vi "10-Tap Conversion.vi"(8 "10 Tap In":T1, 9 "64 Bit In":u64, 10 "16 Bit In":u16, 11 "Operation":T2) -> (1 "10 Tap Out":T1, 2 "64 Bit Out":u64, 3 "16 Bit Out":u16)   [LabVIEW 2013]
uses:
  Common/CL Data to Pixels/10-Tap 8-bit Cluster.ctl
  10-Tap Conversion Enum.ctl
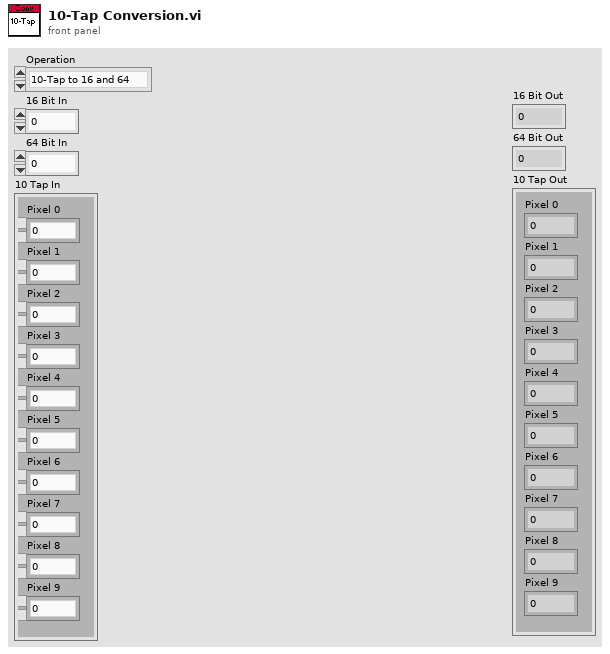
[diagram p1: front panel]
types:
  T1 = typedef "10-Tap 8-bit Cluster.ctl" = cluster{"Pixel 0":u8, "Pixel 1":u8, "Pixel 2":u8, "Pixel 3":u8, "Pixel 4":u8, "Pixel 5":u8, "Pixel 6":u8, "Pixel 7":u8, "Pixel 8":u8, "Pixel 9":u8}
  T2 = typedef "10-Tap Conversion Enum.ctl" = enum16{"10-Tap to 16 and 64", "16 and 64 to 10-Tap"}
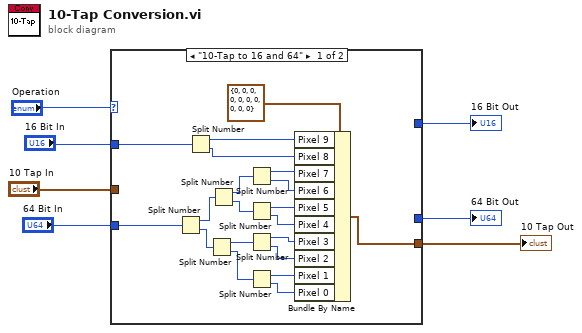
[diagram p0: block diagram]
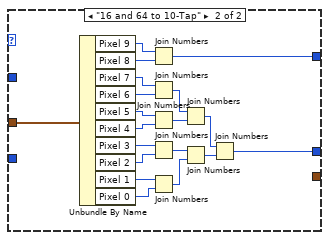
[diagram p2: hidden frame]
diagram:
  n1 = case shown="\"10-Tap to 16 and 64\"" "Operation" {
    tunnel: "10 Tap In" -> [_ w30]
    tunnel: [_ w29] -> w6
    tunnel: [_ w28] -> w5
    tunnel: "16 Bit In" -> [w10 _]
    tunnel: "64 Bit In" -> [w9 _]
    tunnel: [w8 _] -> w1
    frame "10-Tap to 16 and 64" {
      n2 = Split Number(x=w9) -> (hi(x)=w20:u32, lo(x)=w21:u32)
      n3 = Split Number(x=w10) -> (hi(x)=w27:u8, lo(x)=w26:u8)
      n4 = Split Number(x=w21) -> (hi(x)=w24:u16, lo(x)=w25:u16)
      n5 = Split Number(x=w20) -> (hi(x)=w22:u16, lo(x)=w23:u16)
      n6 = Split Number(x=w22) -> (hi(x)=w19:u8, lo(x)=w18:u8)
      n7 = Split Number(x=w23) -> (hi(x)=w17:u8, lo(x)=w16:u8)
      n8 = Split Number(x=w24) -> (hi(x)=w15:u8, lo(x)=w14:u8)
      n9 = Split Number(x=w25) -> (hi(x)=w13:u8, lo(x)=w12:u8)
      n10 = Bundle By Name(cluster=T1 {"Pixel 0"=0, "Pixel 1"=0, "Pixel 2"=0, "Pixel 3"=0, "Pixel 4"=0, "Pixel 5"=0, "Pixel 6"=0, "Pixel 7"=0, "Pixel 8"=0, "Pixel 9"=0} ("10 Tap In"), "Pixel 9"=w27, "Pixel 8"=w26, "Pixel 7"=w19, "Pixel 6"=w18, "Pixel 5"=w17, "Pixel 4"=w16, "Pixel 3"=w15, "Pixel 2"=w14, "Pixel 1"=w13, "Pixel 0"=w12) -> (w8:T1)
    }
    frame "16 and 64 to 10-Tap" {
      n11 = Unbundle By Name(w30) -> ("Pixel 9"=w46:u8, "Pixel 8"=w45:u8, "Pixel 7"=w44:u8, "Pixel 6"=w43:u8, "Pixel 5"=w42:u8, "Pixel 4"=w41:u8, "Pixel 3"=w40:u8, "Pixel 2"=w39:u8, "Pixel 1"=w38:u8, "Pixel 0"=w37:u8)
      n12 = Join Numbers(hi=w46, lo=w45) -> ((hi.lo)=w29:u16)
      n13 = Join Numbers(hi=w44, lo=w43) -> ((hi.lo)=w35:u16)
      n14 = Join Numbers(hi=w42, lo=w41) -> ((hi.lo)=w34:u16)
      n15 = Join Numbers(hi=w40, lo=w39) -> ((hi.lo)=w33:u16)
      n16 = Join Numbers(hi=w38, lo=w37) -> ((hi.lo)=w36:u16)
      n17 = Join Numbers(hi=w35, lo=w34) -> ((hi.lo)=w32:u32)
      n18 = Join Numbers(hi=w33, lo=w36) -> ((hi.lo)=w31:u32)
      n19 = Join Numbers(hi=w32, lo=w31) -> ((hi.lo)=w28:u64)
    }
  }
  "16 Bit Out" <- w6
  "64 Bit Out" <- w5
  "10 Tap Out" <- w1
